vi "tsdb_get_can_db_count.vi"(8 "error in (no error)":errorcluster caption="错误输入（无错误）", 11 "路径输入":path) -> (0 "error out":errorcluster caption="错误输出", 1 "ACount out":i32, 2 "return":i32, 3 "路径输出":path)   [LabVIEW 2014]
doc: "Function Introduction : \nRetrieve the quantity of all loaded LIN databases\nCall location :\ninput parameter :\nACount: Returned database count\nReturn value :\n==0: Execution successful\nOther values: Query error code"
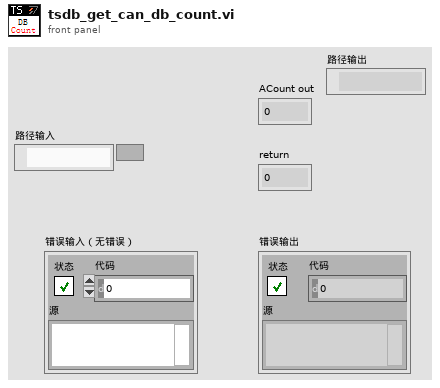
[diagram p1: front panel]
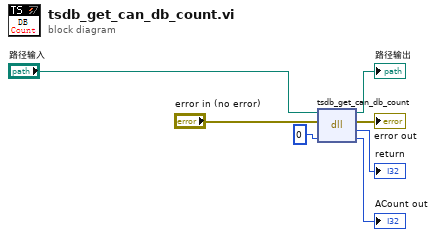
[diagram p0: block diagram]
diagram:
  n1 = dll-call lib="D:/Program Files (x86)/TOSUN/TSMaster/bin/TSMaster.dll" fn="tsdb_get_can_db_count"(path in="路径输入", error in="error in (no error)", "ACount"=0) -> (path out=→"路径输出":path, error out=→"error out":errorcluster, "返回类型"=→"return":i32, "ACount"=→"ACount out":i32)  [unwired: 1 in]
